vi "Z6_Beamline.get data to modify.vi"(0 "i ref in":refnum<vi>, 3 "ms timeout (10000)":i32=10000, 5 "error in (no error)":errorcluster) -> (14 "i ref out":refnum<vi>, 16 "i attribute":T1={"Subs ok GUI Refs"={"Northtower ok"=refnum, "Southtower ok"=refnum, "Frontends ok"=refnum, "100TW COS ok"=refnum}, "Refs BL Northtower"=[], "Refs BL Southtower"=[], "Refs BL 100TW COS"=[], "State Subsystems"={"Northtower"=FALSE, "Southtower"=FALSE, "Frontends"=FALSE, "100TW COS"=FALSE}, "Z6 Beamline Status Subscriber Information"={"BL Z6 Shutter"={"Index of element"=0, "Attributeset"=enum."Boolean Status Service Subscriber"}, "CH 10"={"Index of element"=0, "Attributeset"=enum."Boolean Status Service Subscriber"}, "CH 11"={"Index of element"=0, "Attributeset"=enum."Boolean Status Service Subscriber"}, "ST Flip Cam"={"Index of element"=0, "Attributeset"=enum."Boolean Status Service Subscriber"}, "ST Flip DB"={"Index of element"=0, "Attributeset"=enum."Boolean Status Service Subscriber"}, "BL Z6 Dump"={"Index of element"=0, "Attributeset"=enum."Boolean Status Service Subscriber"}}, "Color State PHELIX"=-1}, 17 "timed out":bool, 19 "error out":errorcluster)   [LabVIEW 2014, in "Z6_Beamline.lvlib"]
doc: "Reads the attribute data of the object after the access to the data has been locked by the \"acquire\" method. If the attribute data has been locked already, this methods waits until the attribute data is unlocked or there is a timeout.\n\nThe attribute data must be unlocked using the methods \"release\" or \"set modified data\".\n\nLicense Agreement for this software:\n\nCopyright (C)\nGesellschaft für Schwerionenforschung, GSI\nPlanckstr. 1\n64291 Darmstadt\nGermany\n\nContact: D.Beck@gsi.de \n\nThis program is free software; you can redistribute it and/or modify it under the terms of the GNU General Public License as published by the Free Software Foundation; either version 2 of the license, or (at your option) any later version.\n\nThis program is distributed in the hope that it will be useful, but WITHOUT ANY WARRANTY; without even the implied warranty of MERCHANTABILITY or FITNESS FOR A PARTICULAR PURPOSE. See the GNU General License for more details (http://www.gnu.org).\n\nGesellschaft für Schwerionenforschung, GSI\nPlanckstr. 1, 64291 Darmstadt, Germany\nFor all questions and ideas contact: M.Richter@gsi.de, H.Brand@gsi.de or D.Beck@gsi.de.\nLast update: 17-JUN-2004"
uses:
  Z6_Beamline.lvlib
  Z6_Beamline.i attribute.ctl
  Z6_Beamline.Subsystem ok GUI Refs.ctl
  Z6_Beamline.Status Subscriber Information.ctl
  PH_BL-Master/PH_BL-Master.Status Subscriber Information.ctl
  PH_BL-Master/PH_BL-Master.Attribute Set.ctl
  CS_Core/CSObj/CSObj.lvlib
  PH_BL-Master/PH_BL-Master.lvlib
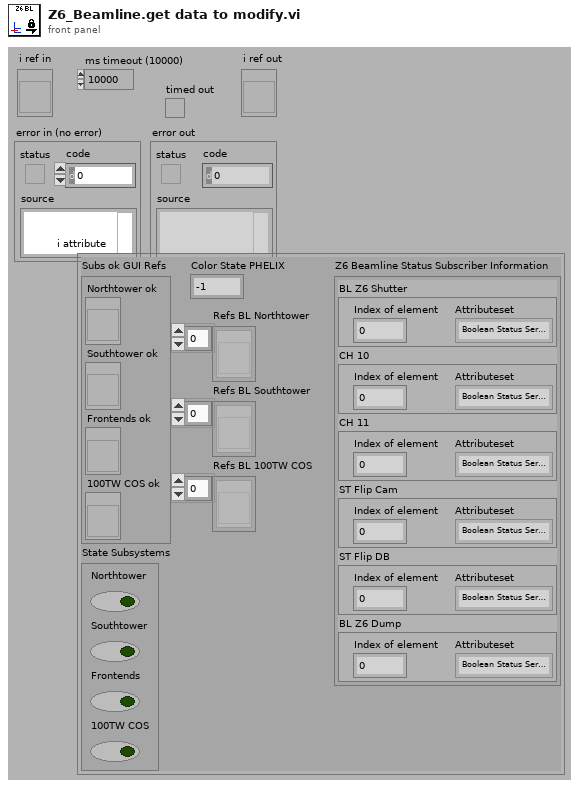
[diagram p1: front panel]
types:
  T1 = typedef "Z6_Beamline.lvlib/Z6_Beamline.i attribute.ctl" = cluster{"Subs ok GUI Refs":T2, "Refs BL Northtower":refnum<vi>[], "Refs BL Southtower":refnum<vi>[], "Refs BL 100TW COS":refnum<vi>[], "State Subsystems":cluster{"Northtower":bool, "Southtower":bool, "Frontends":bool, "100TW COS":bool}, "Z6 Beamline Status Subscriber Information":T3, "Color State PHELIX":i16}
  T2 = typedef "Z6_Beamline.lvlib/Z6_Beamline.Subsystem ok GUI Refs.ctl" = cluster{"Northtower ok":refnum<vi>, "Southtower ok":refnum<vi>, "Frontends ok":refnum<vi>, "100TW COS ok":refnum<vi>}
  T3 = typedef "Z6_Beamline.lvlib/Z6_Beamline.Status Subscriber Information.ctl" = cluster{"BL Z6 Shutter":T4, "CH 10":T4, "CH 11":T4, "ST Flip Cam":T4, "ST Flip DB":T4, "BL Z6 Dump":T4}
  T4 = typedef "PH_BL-Master.lvlib/PH_BL-Master.Status Subscriber Information.ctl" = cluster{"Index of element":i32, "Attributeset":T5}
  T5 = typedef "PH_BL-Master.lvlib/PH_BL-Master.Attribute Set.ctl" = enum16{"Boolean Status Service Subscriber", "Picture Status Service Subscriber"}
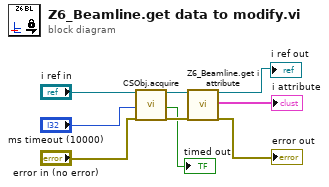
[diagram p0: block diagram]
diagram:
  n1 = call "CSObj.acquire.vi"("i ref in"="i ref in", "ms timeout (10000)"="ms timeout (10000)", "error in (no error)"="error in (no error)") -> ("i ref out"=w8:refnum<vi>, "timed out"=→"timed out":bool, "error out"=w5:errorcluster)  [unwired: 14 in]
  n2 = call "Z6_Beamline.get i attribute.vi"("i ref in"=w8, "error in (no error)"=w5) -> ("i ref out"=→"i ref out":refnum<vi>, "i attribute"=→"i attribute":T1, "error out"=→"error out":errorcluster)  [unwired: 15 in]
